vi "CRYPost Processing Global.vi"() -> ()   [LabVIEW 2013]
panel:
  in  "disp_unit":string
  out "User Equation VI Ref":refnum<vi>
  out "Post Editor VI Ref":refnum<vi>
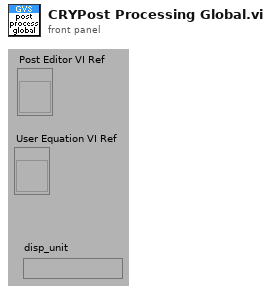
[diagram p1: front panel]
diagram:
